vi "Computer Info.vi"(2 "error in (no error)":errorcluster) -> (0 "error out":errorcluster, 1 "Computer Info":string[][](table))   [LabVIEW 2013]
uses:
  System.Management
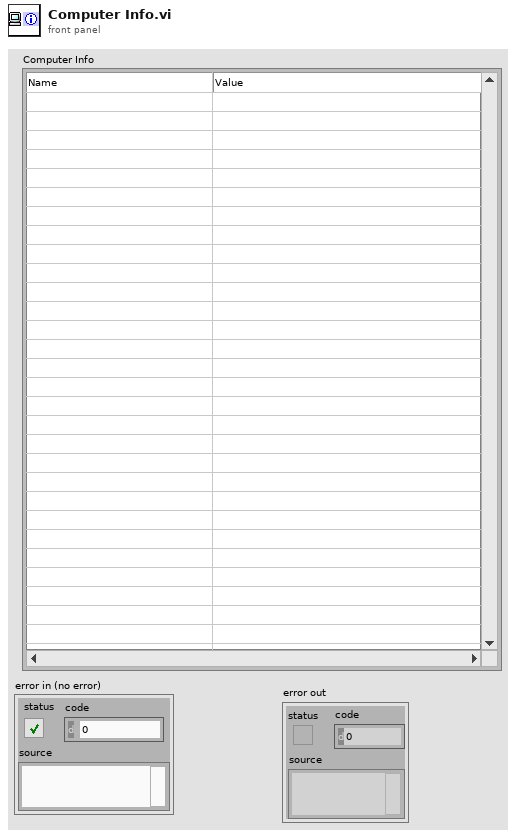
[diagram p1: front panel]
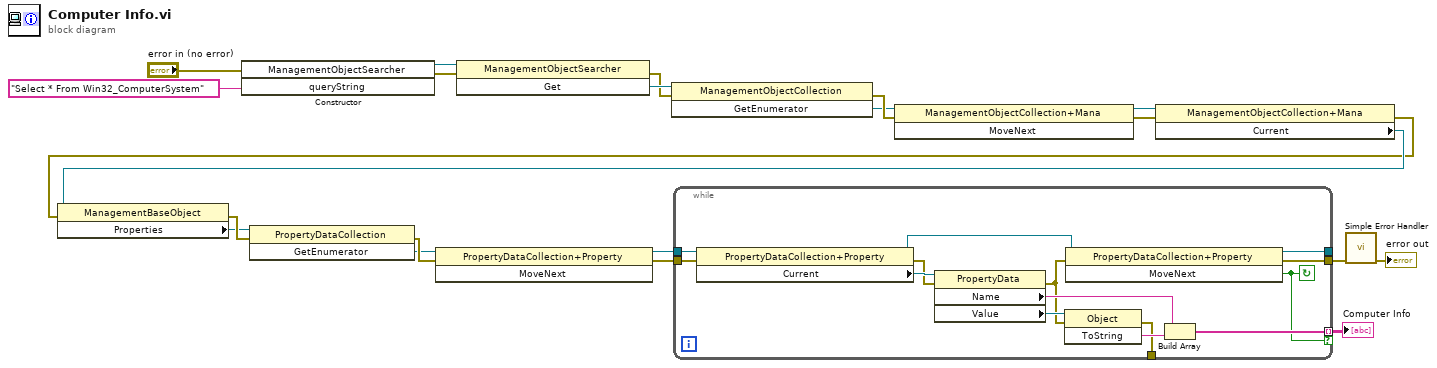
[diagram p0: block diagram]
diagram:
  n1 = constructor class="ManagementObjectSearcher"(error in="error in (no error)", "queryString"="Select * From Win32_ComputerSystem" ("query")) -> (reference out=w17:refnum<k24>, error out=w16:errorcluster)  [unwired: 2 in, 2 out]
  n2 = invoke class="ManagementObjectSearcher" method="Get"(reference=w17, error in=w16) -> (error out=w18:errorcluster, "Get"=w19:refnum<k24>)  [unwired: 1 in, 1 out]
  n3 = invoke class="ManagementObjectCollection" method="GetEnumerator"(reference=w19, error in=w18) -> (error out=w21:errorcluster, "GetEnumerator"=w20:refnum<k24>)  [unwired: 1 in, 1 out]
  n4 = invoke class="ManagementObjectCollection+Mana" method="MoveNext"(reference=w20, error in=w21) -> (reference out=w14:refnum<k24>, error out=w13:errorcluster)  [unwired: 1 in, 1 out]
  n5 = property class="ManagementObjectCollection+Mana"(reference=w14, error in=w13) -> (error out=w4:errorcluster, "Current"=w5:refnum<k24>)  [unwired: 1 out]
  n6 = property class="ManagementBaseObject"(reference=w5, error in=w4) -> (error out=w10:errorcluster, "Properties"=w7:refnum<k24>)  [unwired: 1 out]
  n7 = invoke class="PropertyDataCollection" method="GetEnumerator"(reference=w7, error in=w10) -> (error out=w11:errorcluster, "GetEnumerator"=w8:refnum<k24>)  [unwired: 1 in, 1 out]
  n8 = invoke class="PropertyDataCollection+Property" method="MoveNext"(reference=w8, error in=w11) -> (reference out=w9:refnum<k24>, error out=w12:errorcluster)  [unwired: 1 in, 1 out]
  n9 = while {
    tunnel: w9 -> [w35]
    tunnel: w12 -> [w33]
    tunnel: [w30] -> w3
    tunnel: [w29] -> _
    tunnel: [w25] -> w6 mode=indexing if=w24
    tunnel: [w22] -> _
    stop <- w24 continue-if-true
    n10 = property class="PropertyDataCollection+Property"(reference=w35, error in=w33) -> (reference out=w32:refnum<k24>, error out=w31:errorcluster, "Current"=w34:refnum<k24>)
    n11 = property class="PropertyData"(reference=w34, error in=w31) -> (error out=w23:errorcluster, "Name"=w27:string, "Value"=w28:refnum<k24>)  [unwired: 1 out]
    n12 = invoke class="Object" method="ToString"(reference=w28, error in=w23) -> (error out=w22:errorcluster, "ToString"=w26:string)  [unwired: 1 in, 1 out]
    n13 = invoke class="PropertyDataCollection+Property" method="MoveNext"(reference=w32, error in=w23) -> (reference out=w29:refnum<k24>, error out=w30:errorcluster, "MoveNext"=w24:bool)  [unwired: 1 in]
    n14 = Build Array(w27, w26) -> (w25:string[])
  }
  "Computer Info" <- w6
  n15 = call <vilib>:"Simple Error Handler.vi"("error in (no error)"=w3) -> ("error out"=→"error out":errorcluster)  [unwired: 4 in, 4 out]
